vi "Destroy.vi"(8 "error in (no error)":errorcluster, 11 "Data in":refnum<class "Data.lvclass">) -> (0 "error out":errorcluster)   [LabVIEW 2012, in "MDSplus.lvlib" / "Data.lvclass"]
uses:
  <vilib>/MDSplus/Classes/Data_Class/Data.lvclass
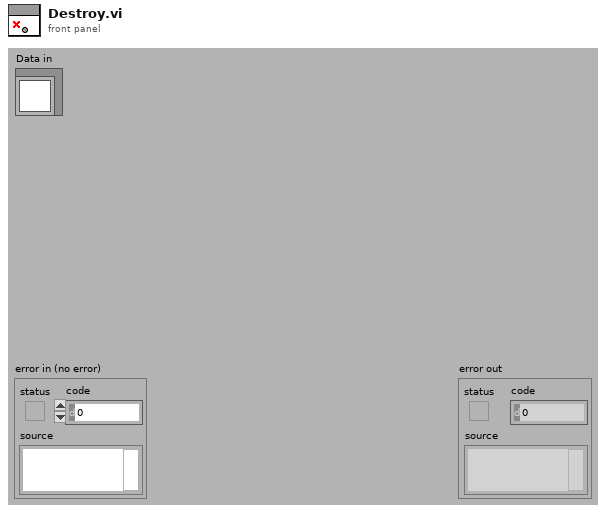
[diagram p1: front panel]
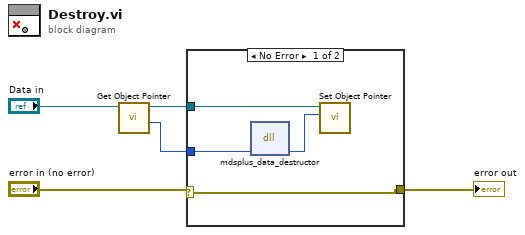
[diagram p0: block diagram]
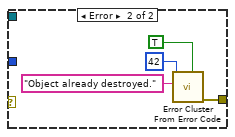
[diagram p2: hidden frame]
diagram:
  n1 = call-dynamic "Get Object Pointer.vi"("Data in"="Data in") -> ("Object Pointer"=w3:i64, "Data out"=w5:refnum<class "Data.lvclass">)  [unwired: 8 in, 1 out]
  n2 = case shown="No Error" "error in (no error)" {
    selector: "error in (no error)" -> [w6 _]
    tunnel: w5 -> [w9 _]
    tunnel: w3 -> [w8 _]
    tunnel: [w6 w11] -> w2
    frame No Error {
      n3 = dll-call lib="MDSobjectsLVShr" fn="mdsplus_data_destructor"("lvDataPtr"=w8) -> ("lvDataPtr"=w7:i64)  [unwired: 4 in, 2 out]
      n4 = call-dynamic "Set Object Pointer.vi"("Object Pointer"=w7, "Data in"=w9) -> ()  [unwired: 9 in, 1 out]
    }
    frame Error {
      n5 = call <vilib>:"Error Cluster From Error Code.vi"("is warning? (False)"=TRUE, "error message (\"\")"="Object already destroyed." ("error message (\"\")"), "error code (0)"=42) -> ("error out"=w11:errorcluster)  [unwired: 6 in]
    }
  }
  "error out" <- w2
